vi "Sand Fall Improved.vi"(4 "Next Possible Locations":cdb[](array[numeric]), 6 "Current Sand Location":cdb, 7 "RockSand Grid in":set{cdb}(c389), 10 "Rock Grid":set{cdb}(c389), 11 "Falling Sand List in":cdb[](array[numeric])) -> (0 "Falling into Void ?":bool, 3 "Falling Sand List out":cdb[](array[numeric]), 5 "RockSand Grid out":set{cdb}(c389))   [LabVIEW 2020, in "AoC 2022.lvlib"]
uses:
  AoC 2022.lvlib
  ede1026b-da77-461f-811e-f3d125b42bc9.vi
  ede1026b-da77-461f-811e-f3d125b42bc9.vi/7c7783df-fd5a-49d9-9b7a-63cc9fb0e4e5.vi
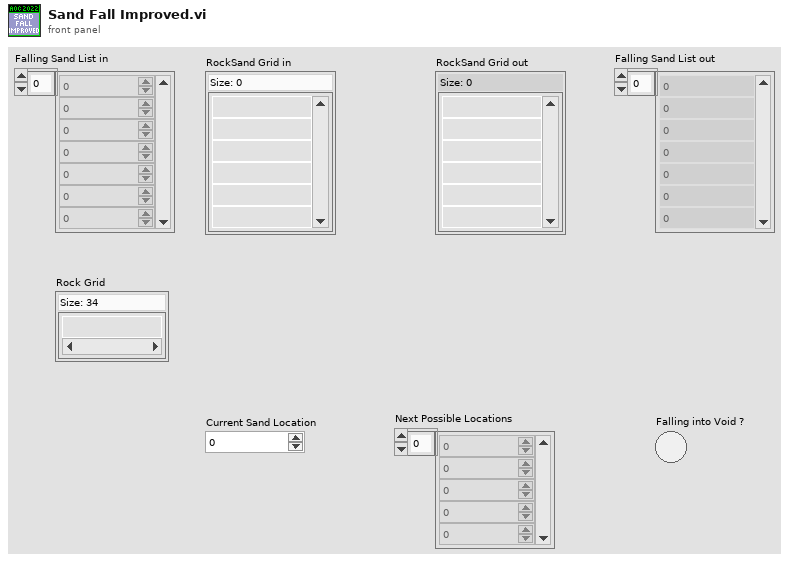
[diagram p1: front panel]
types:
  T1 = cluster{"Left":i16, "Top":i16, "Right":i16, "Bottom":i16}
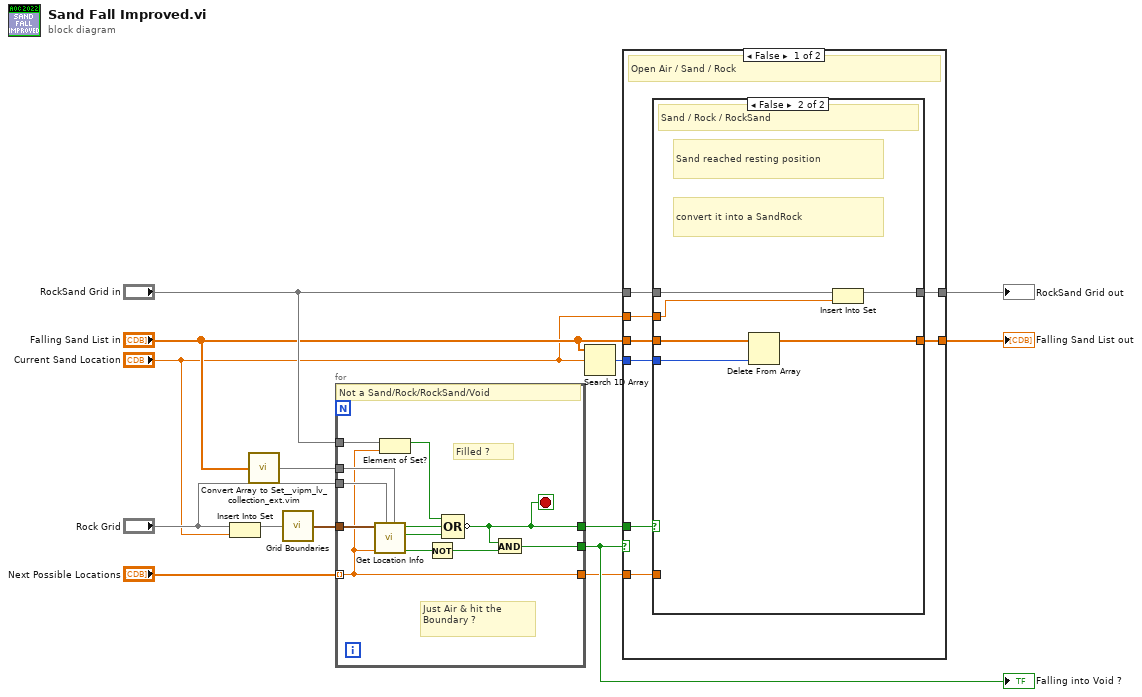
[diagram p0: block diagram]
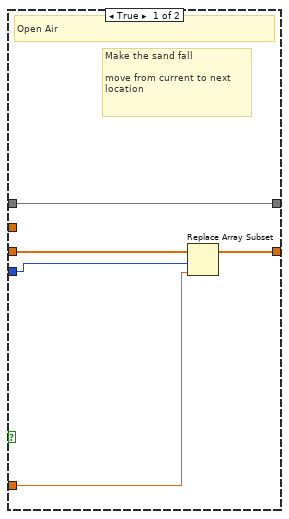
[diagram p2: hidden frame]
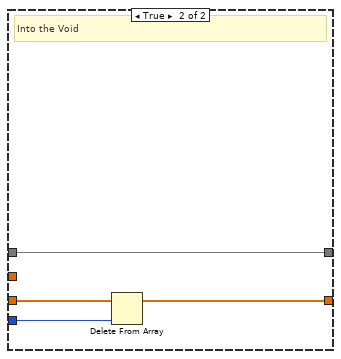
[diagram p3: hidden frame]
diagram:
  n1 = Insert Into Set(10:"Current Sand Location", 11:"Rock Grid") -> (3:w5:set{cdb})  [unwired: 1 out]
  n2 = call "Convert Array to Set__vipm_lv_collection_ext.vim"("array"="Falling Sand List in") -> ("set"=w4:set{cdb})  [unwired: 6 in]
  n3 = call "Grid Boundaries.vi"("Grid"=w5) -> ("Bounds"=w12:T1)
  n4 = for {
    tunnel: [w15] -> w9
    tunnel: [w16] -> w10
    tunnel: w12 -> [w24]
    tunnel: "Rock Grid" -> [w23]
    tunnel: w4 -> [w22]
    tunnel: "Next Possible Locations" -> [w20] mode=indexing
    tunnel: [w20] -> w8
    tunnel: "RockSand Grid in" -> [w21]
    stop <- w15 stop-if-true
    # "Just Air & hit the Boundary ?"
    # "Filled ?"
    # "Not a Sand/Rock/RockSand/Void"
    n5 = call "Get Location Info.vi"("Sand Grid"=w22, "Rock Grid"=w23, "Location"=w20, "Grid Bounds"=w24) -> ("Within the Grid ?"=w25:bool, "Filled with Rock ?"=w26:bool, "Filled with Sand ?"=w17:bool)  [unwired: 3 in]
    n6 = Element of Set?(10:w20, 11:w21) -> (3:w19:bool)
    n7 = Not(x=w25) -> (.not. x?=w18:bool)
    n8 = Compound Arithmetic op=OR(w19, w17, w26) -> (invert w15:bool)
    n9 = And(x=w15, y=w18) -> (x .and. y?=w16:bool)
  }
  "Falling into Void ?" <- w10
  n10 = Search 1D Array(1D array="Falling Sand List in", element="Current Sand Location") -> (index of element=w2:i32)  [unwired: 1 in]
  n11 = case shown="False" w10 {
    tunnel: [w34 w47] -> w14
    tunnel: "Falling Sand List in" -> [w33 w48]
    tunnel: [w31 w49] -> w13
    tunnel: "RockSand Grid in" -> [w30 w49]
    tunnel: w9 -> [w32 _]
    tunnel: w8 -> [w29 _]
    tunnel: w2 -> [w28 w46]
    tunnel: "Current Sand Location" -> [w27 _]
    frame False {
      # "Open Air / Sand / Rock"
      n12 = case shown="False" w32 {
        tunnel: [w37 w42] -> w34
        tunnel: w33 -> [w38 w45]
        tunnel: [w39 w43] -> w31
        tunnel: w30 -> [w39 w44]
        tunnel: w29 -> [w36 _]
        tunnel: w28 -> [w35 w41]
        tunnel: w27 -> [_ w40]
        frame True {
          # "Make the sand fall\n\nmove from current to next location"
          # "Open Air"
          n13 = Replace Array Subset(array=w38, new element=w36, index=w35) -> (w37:cdb[])
        }
        frame False {
          # "convert it into a SandRock"
          # "Sand reached resting position"
          # "Sand / Rock / RockSand"
          n14 = Delete From Array(array=w45, index=w41) -> (array with subset deleted=w42:cdb[])  [unwired: 1 in, 1 out]
          n15 = Insert Into Set(10:w40, 11:w44) -> (3:w43:set{cdb})  [unwired: 1 out]
        }
      }
    }
    frame True {
      # "Into the Void"
      n16 = Delete From Array(array=w48, index=w46) -> (array with subset deleted=w47:cdb[])  [unwired: 1 in, 1 out]
    }
  }
  "Falling Sand List out" <- w14
  "RockSand Grid out" <- w13
